vi "peak - calculate lorentzian - V2.vi"(8 "4corners":T1={"z (-pi/2)"=-1.0311345636926572+0.5736824521422934i, "z(inf)"=-0.5200164984937075+1.0975277942502903i, "z (pi/2)"=-1.0311345636926572+0.5736824521422934i, "z center"=-0.5136528600391839+0.580046090596817i, "z(0)"=-0.5200164984937075+1.0975277942502903i, "radius"=-1.0311345636926572}, 10 "gamma":dbl, 11 "omega":dbl) -> (3 "lorentzian out":T2={"Amplitude"=-1.0311345636926572, "omega(0)"=-1.0311345636926572, "Gamma"=-1.0311345636926572, "phase"=-1.0311345636926572, "Q"=-1.0311345636926572, "Norm  Ampl"=-1.0311345636926572, "z (inf)"=-1.0311345636926572+0.0i, "4corners"={"z (-pi/2)"=-1.0311345636926572+0.5736824521422934i, "z(inf)"=-0.5200164984937075+1.0975277942502903i, "z (pi/2)"=-1.0311345636926572+0.5736824521422934i, "z center"=-0.5136528600391839+0.580046090596817i, "z(0)"=-0.5200164984937075+1.0975277942502903i, "radius"=-1.0311345636926572}} {"z (inf)" format="%#9_9f"; "Q" format="%#9_9f"; "phase" format="%#9_9f"; "Gamma" format="%#9_9f"; "omega(0)" format="%#9_9f"})   [LabVIEW 2010]
uses:
  lorentzian.ctl
  circle corners.ctl
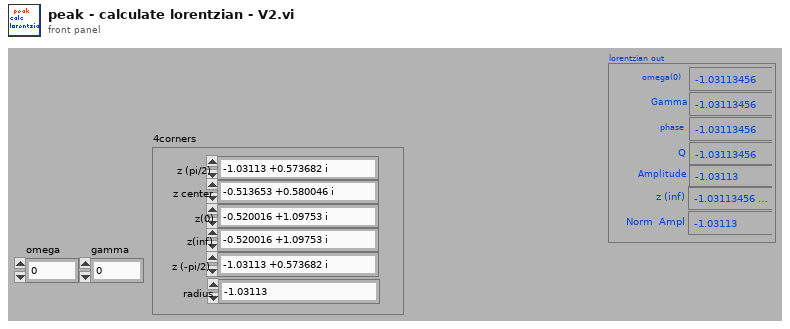
[diagram p1: front panel]
types:
  T1 = typedef "circle corners.ctl" = cluster{"z (-pi/2)":cdb, "z(inf)":cdb, "z (pi/2)":cdb, "z center":cdb, "z(0)":cdb, "radius":dbl}
  T2 = typedef "lorentzian.ctl" = cluster{"Amplitude":dbl, "omega(0)":dbl, "Gamma":dbl, "phase":dbl, "Q":dbl, "Norm  Ampl":dbl, "z (inf)":cdb, "4corners":T1}
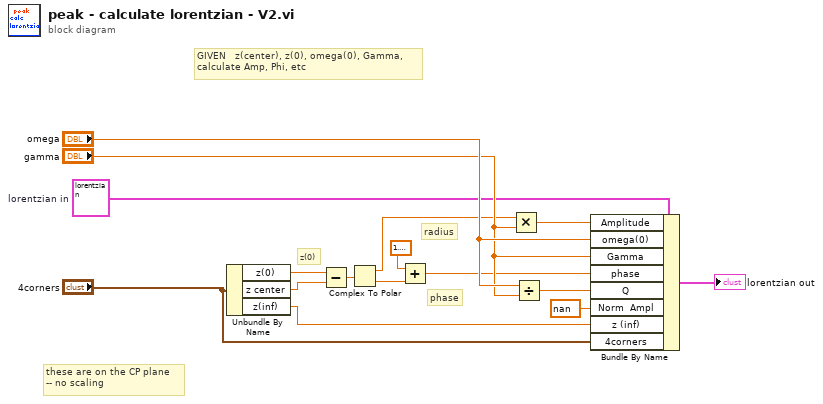
[diagram p0: block diagram]
diagram:
  w12 = T2 {"Amplitude"=0.0, "omega(0)"=0.0, "Gamma"=0.0, "phase"=0.0, "Q"=0.0, "Norm  Ampl"=0.0, "z (inf)"=0.0+0.0i, "4corners"={"z (-pi/2)"=0.0+0.0i, "z(inf)"=0.0+0.0i, "z (pi/2)"=0.0+0.0i, "z center"=0.0+0.0i, "z(0)"=0.0+0.0i, "radius"=0.0}}  # lorentzian in
  # "these are on the CP plane \n-- no scaling"
  # "z(0)"
  # "radius"
  # "phase"
  # "GIVEN   z(center), z(0), omega(0), Gamma, \ncalculate Amp, Phi, etc"
  n1 = Unbundle By Name("4corners") -> ("z(0)"=w1:cdb, "z center"=w11:cdb, "z(inf)"=w10:cdb)
  n2 = Subtract(x=w1, y=w11) -> (x-y=w9:cdb)
  n3 = Complex To Polar(r * e^(i*theta)=w9) -> (r=w4:dbl, theta=w7:dbl)
  n4 = Add(x=1.5707963267948966, y=w7) -> (x+y=w6:dbl)
  n5 = Multiply(x=w4, y="gamma") -> (x*y=w3:dbl)
  n6 = Divide(x="omega", y="gamma") -> (x/y=w5:dbl)
  n7 = Bundle By Name(cluster=w12, "Amplitude"=w3, "omega(0)"="omega", "Gamma"="gamma", "phase"=w6, "Q"=w5, "Norm  Ampl"=nan, "z (inf)"=w10, "4corners"="4corners") -> (→"lorentzian out":T2)
